vi "KH TURCK ETHERNETIP FGlob RFID TAG0 AO.vi"(6 "Nr Module":i32, 7 "Function":T1=enum."Recall one", 8 "err in":errorcluster caption="error", 10 "RFID one in":u8[](array[numeric]), 11 "RFID all in":u8[](array[numeric])) -> (0 "err out":errorcluster caption="error", 2 "RFID one out":u8[](array[numeric]), 3 "RFID all out":u8[](array[numeric]))   [LabVIEW 2021]
uses:
  KH TURCK TypeDefs FGlob.ctl
  KH TURCK ETHERNETIP RFID Global.vi
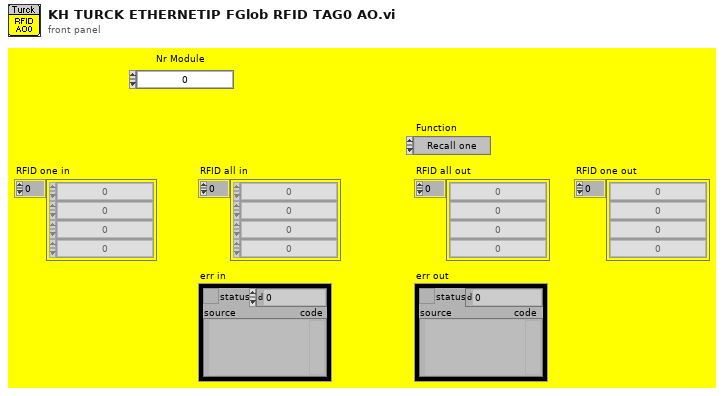
[diagram p1: front panel]
types:
  T1 = typedef "KH TURCK TypeDefs FGlob.ctl" = enum16{"Put one", "Put all", "Recall one", "Recall all"}
  T2 = typedef "KH TURCK ETHERNETIP TDefCluster TURCK RFID.ctl" = cluster{"NumberOfBytes":i32, "State":string, "Counter":i32, "ReadData":u8[], "AnzahlFragmente":i32, "WritingFinished":bool, "ReadingFinished":bool, "UID":u8[], "ActCommand":T3, "SizeFragmentRead":i32, "LengthUID":u16, "WriteDataInclUID":u8[], "Timeout":bool, "SizeFragmentWrite":i32}
  T3 = typedef "KH TURCK ETHERNETIP TDef Enum RFID Act Command.ctl" = enum16{"read", "write", "idle", "Inventory", ""}
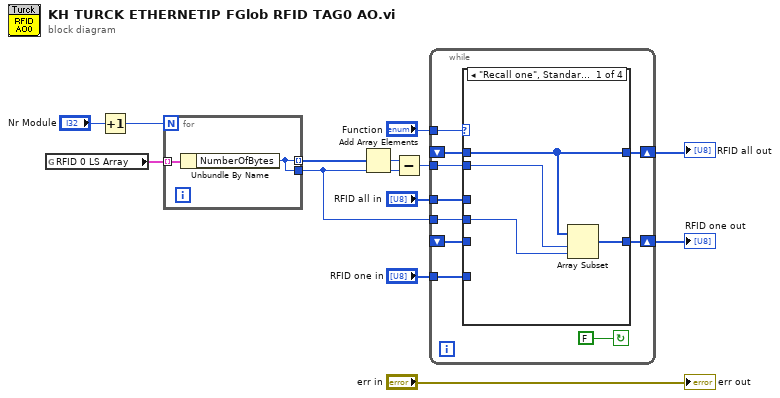
[diagram p0: block diagram]
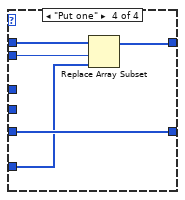
[diagram p4: hidden frame]
diagram:
  n1 = global read "KH TURCK ETHERNETIP RFID Global.vi" "RFID 0 LS Array"() -> (w7:T2[])
  n2 = Increment(x="Nr Module") -> (x+1=w1:i32)
  n3 = for {
    N: w1 -> [_]
    tunnel: w7 -> [w15] mode=indexing
    tunnel: [w14] -> w6 mode=indexing
    tunnel: [w14] -> w3
    n4 = Unbundle By Name(w15) -> ("NumberOfBytes"=w14:i32)
  }
  n5 = Add Array Elements(numeric array=w6) -> (sum=w5:i32)
  n6 = Subtract(x=w5, y=w3) -> (x-y=w4:i32)
  n7 = while {
    shift-right: [w23] -> w11
    shift-left: _ -> [w22]
    tunnel: "Function" -> [w24]
    tunnel: w4 -> [w20]
    tunnel: "RFID all in" -> [w19]
    shift-right: [w21] -> w8
    shift-left: _ -> [w18]
    tunnel: "RFID one in" -> [w17]
    tunnel: w3 -> [w16]
    stop <- FALSE continue-if-true
    n8 = case shown="\"Recall one\", Standard" w24 {
      tunnel: [w29 w31 w32 w36] -> w23
      tunnel: w22 -> [w29 w31 _ w37]
      tunnel: w20 -> [w28 _ _ w38]
      tunnel: [w27 w30 w33 w35] -> w21
      tunnel: w19 -> [_ _ w32 _]
      tunnel: w18 -> [_ w30 w33 w35]
      tunnel: w17 -> [_ _ _ w34]
      tunnel: w16 -> [w26 _ _ _]
      frame "Recall one", Default {
        n9 = Array Subset(array=w29, index=w28, length=w26) -> (w27:u8[])
      }
      frame "Recall all" {
      }
      frame "Put all" {
      }
      frame "Put one" {
        n10 = Replace Array Subset(array=w37, new element=w34, index=w38) -> (w36:u8[])
      }
    }
  }
  "RFID all out" <- w11
  "RFID one out" <- w8
  "err out" <- "err in"
